vi "Close vi references.vi"(11 "map":map{string, refnum<vi>}(c390)) -> ()   [LabVIEW 2020, in "Dashboard.lvlib"]
uses:
  Dashboard.lvlib
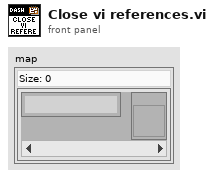
[diagram p1: front panel]
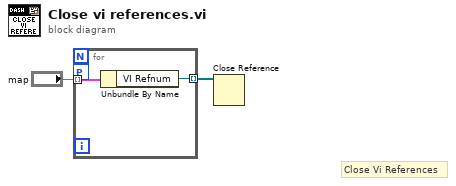
[diagram p0: block diagram]
diagram:
  # "Close Vi References"
  n1 = for {
    tunnel: "map" -> [w4] mode=indexing
    tunnel: [w3] -> w2 mode=indexing
    workers-P: _ -> [_]
    n2 = Unbundle By Name(w4) -> ("VI Refnum"=w3:refnum<vi>)
  }
  n3 = Close Reference(reference=w2) -> ()  [unwired: 1 in, 1 out]
